vi "SLSC SPI Engine.vi"(8 "error in (no error)":errorcluster, 10 "SPI API References":T2, 11 "Chip Select DIO Lines":T1={"SCLK"="Port0/DIO3", "MISO"="Port0/DIO3", "MOSI"="Port0/DIO3", "CS 0"="Port0/DIO3", "CS 1"="Port0/DIO4", "CS 2"="Port0/DIO4", "CS 3"="Port0/DIO1", "CS 4"="Port0/DIO4", "CS 5"="Port0/DIO4"}) -> ()   [LabVIEW 2014, in "SLSC FPGA Toolkit.lvlib"]
uses:
  <vilib>/SPI API/SPIAPI/Controls/Internal Data (SPI API).ctl
  <vilib>/SPI API/SPIAPI/DIO/SPI Digital IO Lines.ctl
  <vilib>/Platform/TimedLoop/XDataNode/timing_clust.ctl
  <vilib>/Platform/TimedLoop/XDataNode/nitl_modes.ctl
  <vilib>/Platform/TimedLoop/XDataNode/wakeup.ctl
  <vilib>/rvi/Emulation/niFpgaSctlEmulationGetInTimedLoop.vi
  <vilib>/rvi/Emulation/niFpgaEmulationReportErrorSimple.vi
  <vilib>/rvi/Emulation/niFpgaGetClockAttributes.vi
  <vilib>/rvi/Emulation/niFpgaCriticalErrorInLSC.vi
  <vilib>/Platform/TimedLoop/XDataNode/XDataNode.xnode
  SLSC FPGA Toolkit.lvlib
  <vilib>/Platform/TimedLoop/XDataNode/XDNodeRunTimeDep.lvlib
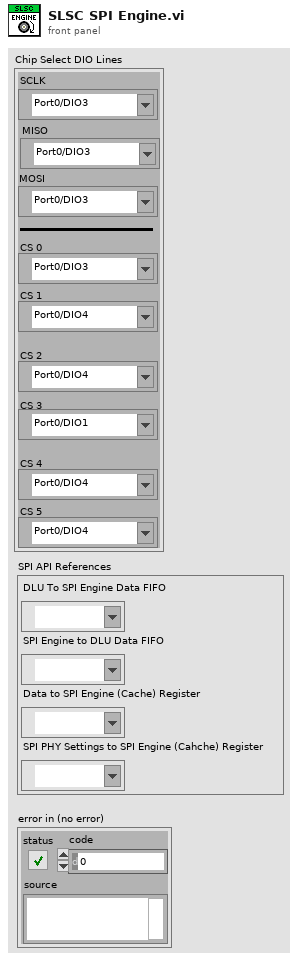
[diagram p1: front panel]
types:
  T1 = typedef "SPI Digital IO Lines.ctl" = cluster{"SCLK":refnum<k21>, "MISO":refnum<k21>, "MOSI":refnum<k21>, "CS 0":refnum<k21>, "CS 1":refnum<k21>, "CS 2":refnum<k21>, "CS 3":refnum<k21>, "CS 4":refnum<k21>, "CS 5":refnum<k21>}
  T2 = typedef "Internal Data (SPI API).ctl" = cluster{"DLU To SPI Engine Data FIFO":refnum<k21>, "SPI Engine to DLU Data FIFO":refnum<k21>, "Data to SPI Engine (Cache) Register":refnum<k21>, "SPI PHY Settings to SPI Engine (Cahche) Register":refnum<k21>}
  T3 = typedef "XDNodeRunTimeDep.lvlib/timing_clust.ctl" = cluster{"Expected End [f-1]":u64, "Actual End [f-1]":u64, "Finished Late? [f-1]":bool, "Expected End [i-1]":u64, "Actual End [i-1]":u64, "Finished Late? [i-1]":bool, "Expected Start [i]":u64, "Actual Start [i]":u64, "Expected Start [f]":u64, "Actual Start [f]":u64, "Source Name":string, "Structure Name":string, "Period":i64, "Deadline":i64, "Offset":i64, "Start":i64, "Priority":i32, "Timeout":i32, "Mode":T4, "Wakeup Reason":T5, "Error":errorcluster, "Source Type":string, "Secondary Source Type":string, "Global End Time":u64, "Global Start Time":u64, "Frame Duration":u64, "Iteration Duration":u64, "Assigned CPU":i32, "I/O Scan Engine Mode":u32}
  T4 = typedef "XDNodeRunTimeDep.lvlib/nitl_modes.ctl" = enum32{"No Change", "Process missed periods, maintain original phase", "Discard missed periods, maintain original phase", "Process missed periods, ignore original phase", "Discard missed periods, ignore original phase"}
  T5 = typedef "XDNodeRunTimeDep.lvlib/wakeup.ctl" = enum32{"Normal", "Aborted", "Asynchronous wakeup", "Timing source error", "Timed loop error", "Timeout"}
  T6 = typedef "NI SPI IP FPGA.lvlib/Spi Master Inputs.ctl" = cluster{"MISO":bool}
  T7 = typedef "NI SPI IP FPGA.lvlib/Spi Master Outputs.ctl" = cluster{"Chip Select":bool, "Clock":bool, "MOSI":bool, "MOSI OE":bool}
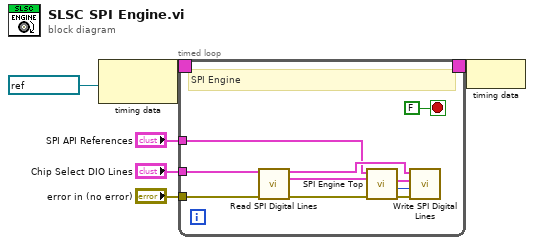
[diagram p0: block diagram]
diagram:
  n1 = node-c288(refnum<k21> "120MHz" ("Source Name")) -> (w6:T3)
  n2 = timed-loop {
    tunnel: "SPI API References" -> [w13]
    tunnel: "error in (no error)" -> [w11]
    tunnel: "Chip Select DIO Lines" -> [w15]
    timing: w6 -> [_]
    timing-out: [_] -> w5
    stop <- FALSE stop-if-true
    # "SPI Engine"
    n3 = call <vilib>:"Read SPI Digital Lines.vi"("Chip Select DIO Lines"=w15, "error in"=w11) -> ("Chip Select DIO Lines Out"=w16:T1, "SPI Read Data"=w12:T6, "error out"=w10:errorcluster)  [unwired: 11 in]
    n4 = call <vilib>:"SPI Engine Top.vi"("error in"=w10, "SPI Read Data"=w12, "SPI API References"=w13) -> ("error out"=w9:errorcluster, "Chip Select ID"=w8:u8, "SPI DIO Output"=w14:T7)  [unwired: 5 in, 1 out]
    n5 = call <vilib>:"Write SPI Digital Lines.vi"("error in"=w9, "CS Index"=w8, "spi output"=w14, "Chip Select DIO Lines"=w16) -> ()  [unwired: 6 in, 2 out]
  }
  n6 = node-c288(w5) -> ()
